vi "Configure DVM Setting.vi"(8 "error in (no error)":errorcluster, 10 "DVM Setting":T1={"DVM Channel"=1, "Enable DVM Analysis"=FALSE, "Auto Range "=FALSE, "DVM Type"=0} {"DVM Type" items=["Root-mean-square, without DC", "DC Value", "Root-mean-square", "Frequency Counter"]; "DVM Channel" items=["Channel 1"=1, "Channel 2"=2, "Channel 3"=3, "Channel 4"=4]}, 11 "Agilent 3054A in":refnum<class "Agilent 3054A.lvclass">) -> (0 "error out":errorcluster, 3 "Agilent 3054A out":refnum<class "Agilent 3054A.lvclass">)   [LabVIEW 2016, in "Oscilloscope.lvlib" / "Agilent 3054A.lvclass"]
uses:
  Agilent 3054A.lvclass
  Agilent 3054A.lvclass/Agilent 3054A.ctl
  <instrlib>/Agilent 2000 3000 X-Series/Agilent 2000 3000 X-Series.lvlib
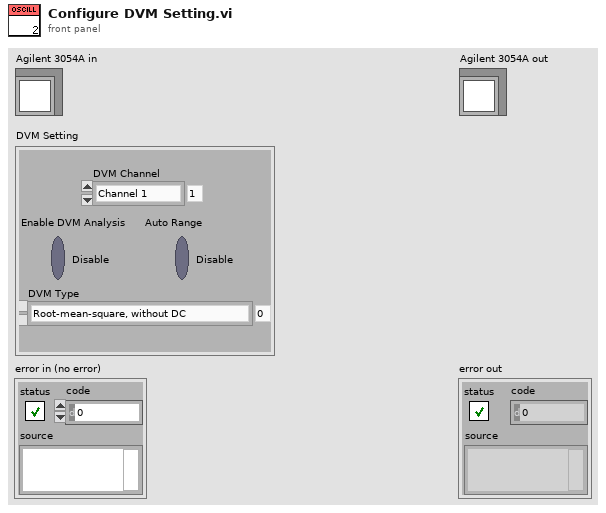
[diagram p1: front panel]
types:
  T1 = cluster{"DVM Channel":i32, "Enable DVM Analysis":bool, "Auto Range ":bool, "DVM Type":i32}
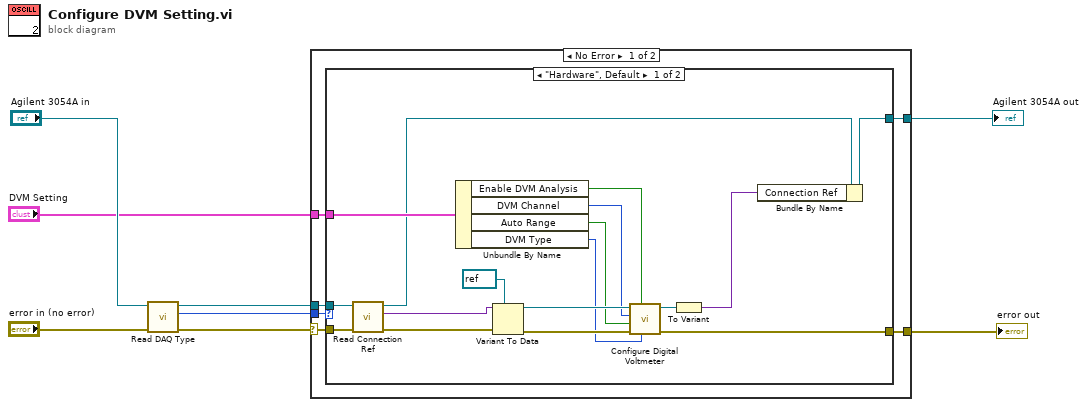
[diagram p0: block diagram]
diagram:
  n1 = call-dynamic "Read DAQ Type.vi"("error in (no error)"="error in (no error)", "Agilent 3054A in"="Agilent 3054A in") -> ("error out"=w7:errorcluster, "DAQ Type"=w6:enum16{"Hardware", "Simulation"}, "Agilent 3054A out"=w5:refnum<class "Agilent 3054A.lvclass">)  [unwired: 7 in]
  n2 = case shown="No Error" w7 {
    selector: w7 -> [w13 w35]
    tunnel: w6 -> [w14 _]
    tunnel: w5 -> [w12 w34]
    tunnel: [w11 w35] -> w4
    tunnel: [w10 w34] -> w3
    tunnel: "DVM Setting" -> [w9 _]
    frame No Error {
      n3 = case shown="\"Hardware\", Default" w14 {
        tunnel: w13 -> [w31 w33]
        tunnel: w12 -> [w30 w32]
        tunnel: [w25 w33] -> w11
        tunnel: [w18 w32] -> w10
        tunnel: w9 -> [w23 _]
        frame "Hardware", Default {
          n4 = call-dynamic "Read Connection Ref.vi"("error in (no error)"=w31, "Agilent 3054A in"=w30) -> ("error out"=w29:errorcluster, "Connection Ref"=w28:variant, "Agilent 3054A out"=w15:refnum<class "Agilent 3054A.lvclass">)  [unwired: 7 in]
          n5 = Unbundle By Name(w23) -> ("Enable DVM Analysis"=w22:bool, "DVM Channel"=w21:i32, "Auto Range"=w20:bool, "DVM Type"=w19:i32)
          n6 = Variant To Data(error in=w29, type=refnum<visa-resource-name> refnum ("VISA resource name"), Variant=w28) -> (data=w24:refnum<visa-resource-name>, error out=w26:errorcluster)
          n7 = call <instrlib>:"Configure Digital Voltmeter.vi"("DVM Type (0: Root-mean-square, without DC)"=w19, "Enable DVM Analysis (F: Disable)"=w22, "error in (no error)"=w26, "Auto Range (F: Disable)"=w20, "DVM Channel (1: Channel 1)"=w21, "VISA resource name"=w24) -> ("error out"=w25:errorcluster, "VISA resource name out"=w17:refnum<visa-resource-name>)  [unwired: 4 in]
          n8 = To Variant(anything=w17) -> (Variant=w16:variant)
          n9 = Bundle By Name(cluster=w15, "Connection Ref"=w16) -> (w18:refnum<class "Agilent 3054A.lvclass">)
        }
        frame "Simulation" {
        }
      }
    }
    frame Error {
    }
  }
  "error out" <- w4
  "Agilent 3054A out" <- w3
